vi "Serial_Transmision_Read_and_Write.vi"(8 "Command":u8=1 min=1 max=1, 9 "Array":u16[](array[numeric]), 10 "error in":errorcluster, 11 "VISA Refnum in":refnum<visa-resource-name>="COM1") -> (0 "unsigned byte array":u8[](array[numeric]), 1 "Command Echo":u8[](array[numeric]), 2 "askii Characters":string, 3 "read buffer":string, 4 "error?":bool, 5 "Transmision uint8 array":u8[](array[numeric]), 6 "Transmision Data in Hex":u8[](array[numeric]) format="%x", 7 "return count":u32)   [LabVIEW 2012]
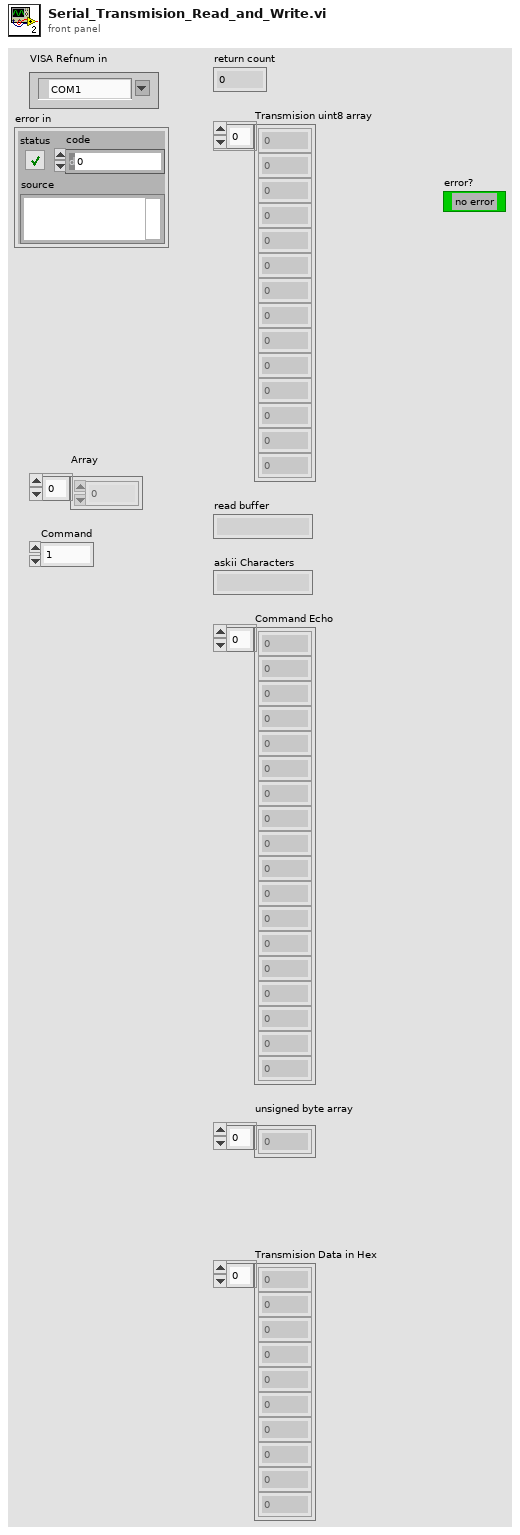
[diagram p1: front panel]
types:
  T1 = cluster{"Packet_Size":u8, "command":u8, "buffer":u8[]}
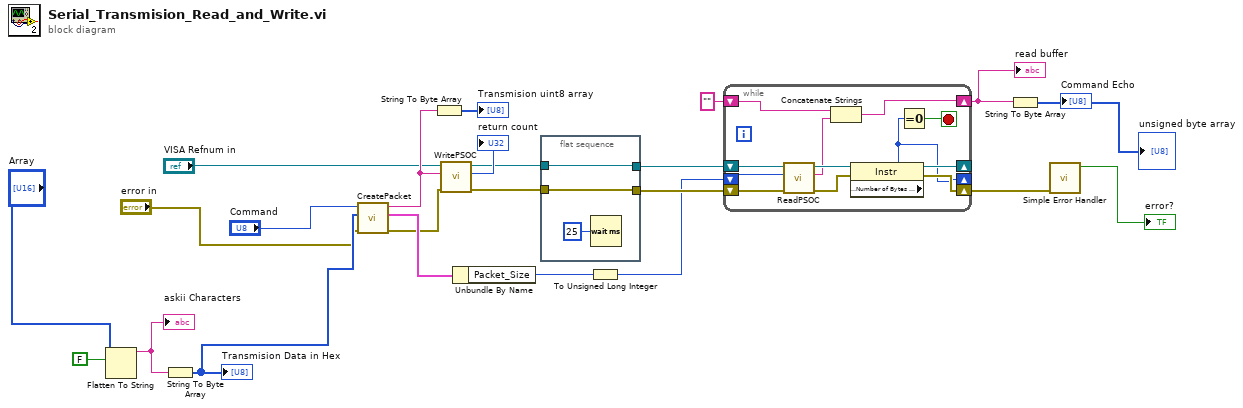
[diagram p0: block diagram]
diagram:
  n1 = Flatten To String(anything="Array", prepend array or string size? (T)=FALSE) -> (data string=w19:string)  [unwired: 2 in, 2 out]
  "askii Characters" <- w19
  n2 = String To Byte Array(string=w19) -> (unsigned byte array=w21:u8[])
  "Transmision Data in Hex" <- w21
  n3 = call "CreatePacket.vi"("error in"="error in", "data"=w21, "command"="Command") -> ("error out"=w5:errorcluster, "output cluster"=w8:T1, "Command String"=w14:string)  [unwired: 6 in]
  n4 = String To Byte Array(string=w14) -> (unsigned byte array=→"Transmision uint8 array":u8[])
  n5 = call "WritePSOC.vi"("error in"=w5, "write buffer"=w14, "VISA resource name"="VISA Refnum in") -> ("error out"=w11:errorcluster, "return count"=→"return count":u32, "VISA resource name out"=w6:refnum<visa-resource-name>)  [unwired: 5 in]
  n6 = Unbundle By Name(w8) -> ("Packet_Size"=w9:u8)
  n7 = flat-sequence {
    tunnel: w6 -> [w26]
    tunnel: [w26] -> w7
    tunnel: [w24] -> w12
    tunnel: w11 -> [w24]
    frame #0 {
      n8 = Wait (ms)(milliseconds to wait=u32 25) -> ()  [unwired: 1 out]
    }
  }
  n9 = To Unsigned Long Integer(number=w9) -> (unsigned 32bit integer=w10:u32)
  n10 = while {
    shift-right: [w34] -> _
    shift-left: w7 -> [w38]
    shift-right: [w32] -> w1
    shift-left: w12 -> [w36]
    shift-right: [w29] -> w17
    shift-left: "" -> [w28]
    shift-right: [w27] -> _
    shift-left: w10 -> [w37]
    stop <- w31 stop-if-true
    n11 = call "ReadPSOC.vi"("error in"=w36, "byte count"=w37, "VISA resource name"=w38) -> ("error out"=w33:errorcluster, "read buffer"=w30:string, "VISA resource name out"=w35:refnum<visa-resource-name>)  [unwired: 5 in]
    n12 = Concatenate Strings(w28, w30) -> (w29:string)
    n13 = property class="Instr"(reference=w35, error in=w33) -> (reference out=w34:refnum<visa-resource-name>, error out=w32:errorcluster, "Serial Settings:Number of Bytes at Serial Port"=w27:u32)
    n14 = Equal To 0?(x=w27) -> (x = 0?=w31:bool)
  }
  "read buffer" <- w17
  n15 = String To Byte Array(string=w17) -> (unsigned byte array=→"Command Echo" →"unsigned byte array":u8[])
  n16 = call <vilib>:"Simple Error Handler.vi"("error in (no error)"=w1) -> ("error?"=→"error?":bool)  [unwired: 4 in, 4 out]
